vi "Write Mutation Delta.vi"(8 "error in (no error)":errorcluster, 10 "Mutation Delta":cluster{"Upper":dbl, "Lower":dbl}, 11 "Real Mutator in":refnum<class "Real Mutator.lvclass">) -> (0 "error out":errorcluster, 3 "Real Mutator out":refnum<class "Real Mutator.lvclass">)   [LabVIEW 2016, in "Real Mutator.lvclass"]
uses:
  Real Mutator.lvclass
  Real Mutator.lvclass/Real Mutator.ctl
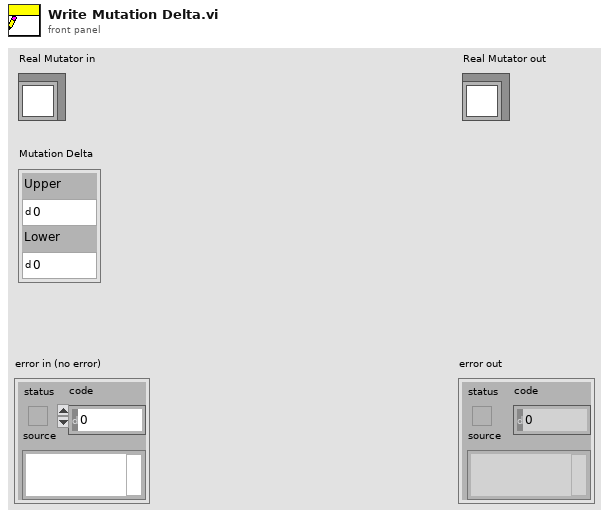
[diagram p1: front panel]
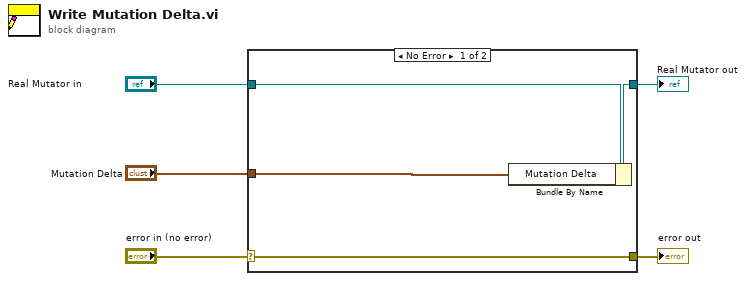
[diagram p0: block diagram]
diagram:
  n1 = case shown="No Error" "error in (no error)" {
    selector: "error in (no error)" -> [w9 w10]
    tunnel: [w9 w10] -> w4
    tunnel: [w7 w11] -> w2
    tunnel: "Real Mutator in" -> [w8 w11]
    tunnel: "Mutation Delta" -> [w6 _]
    frame No Error {
      n2 = Bundle By Name(cluster=w8, "Mutation Delta"=w6) -> (w7:refnum<class "Real Mutator.lvclass">)
    }
    frame Error {
    }
  }
  "error out" <- w4
  "Real Mutator out" <- w2
